vi "Get Picture.vi"(8 "error in (no error)":errorcluster, 11 "Wooden Case in":refnum<class "Wooden Case.lvclass">) -> (0 "error out":errorcluster, 2 "Picture":picture, 3 "Wooden Case out":refnum<class "Wooden Case.lvclass">)   [LabVIEW 2020, in "Wooden Case.lvclass"]
uses:
  Wooden Case.lvclass
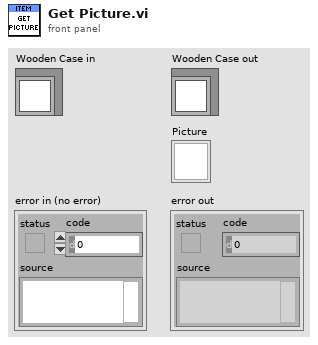
[diagram p1: front panel]
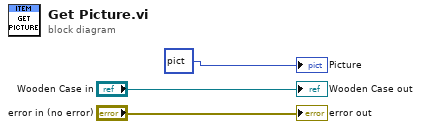
[diagram p0: block diagram]
diagram:
  "error out" <- "error in (no error)"
  "Wooden Case out" <- "Wooden Case in"
  "Picture" <- picture bytes[3230] ("new picture")
